vi "Error Message display(condition wise).vi"(6 "Check Status(2-hi,1Lo,0 def":u8=2, 7 "Index No":i32, 8 "Signal Lo Message":string[](array[string]), 9 "Signal Hi Message":string[](array[string])) -> (2 "Message":string)   [LabVIEW 2015]
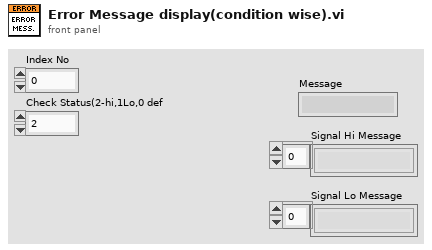
[diagram p1: front panel]
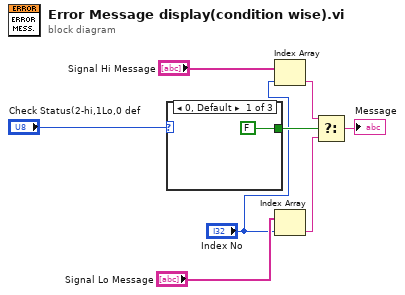
[diagram p0: block diagram]
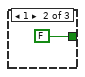
[diagram p2: hidden frame]
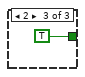
[diagram p3: hidden frame]
diagram:
  n1 = case shown="0, Default" "Check Status(2-hi,1Lo,0 def" {
    tunnel: [FALSE ("f") FALSE ("f") TRUE ("f")] -> w7
    frame 0, Default {
    }
    frame 1 {
    }
    frame 2 {
    }
  }
  n2 = Index Array(array="Signal Hi Message", index="Index No") -> (element=w5:string)
  n3 = Index Array(array="Signal Lo Message", index="Index No") -> (element=w2:string)
  n4 = Select(t=w5, s=w7, f=w2) -> (s? t:f=→"Message":string)
